vi "bullet amount.vi"() -> ()   [LabVIEW 2025]
panel:
  out "Bullet amount":u32
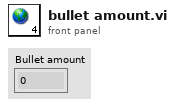
[diagram p1: front panel]
diagram:
